vi "test_count2.vi"() -> ()   [LabVIEW 2013]
uses:
  <instrlib>/_niInstr/Basic Elements/v1/FPGA/Private/Count Down U32.vi
  <instrlib>/_niInstr/Basic Elements/v1/FPGA/niInstr Basic Elements v1 FPGA.lvlib
panel:
  out "Waveform Graph 4":i16[][](graph)
  out "Waveform Graph 3":i16[][](graph)
  out "Waveform Graph 2":u32[](graph)
  out "counting":bool
  out "output valid":bool
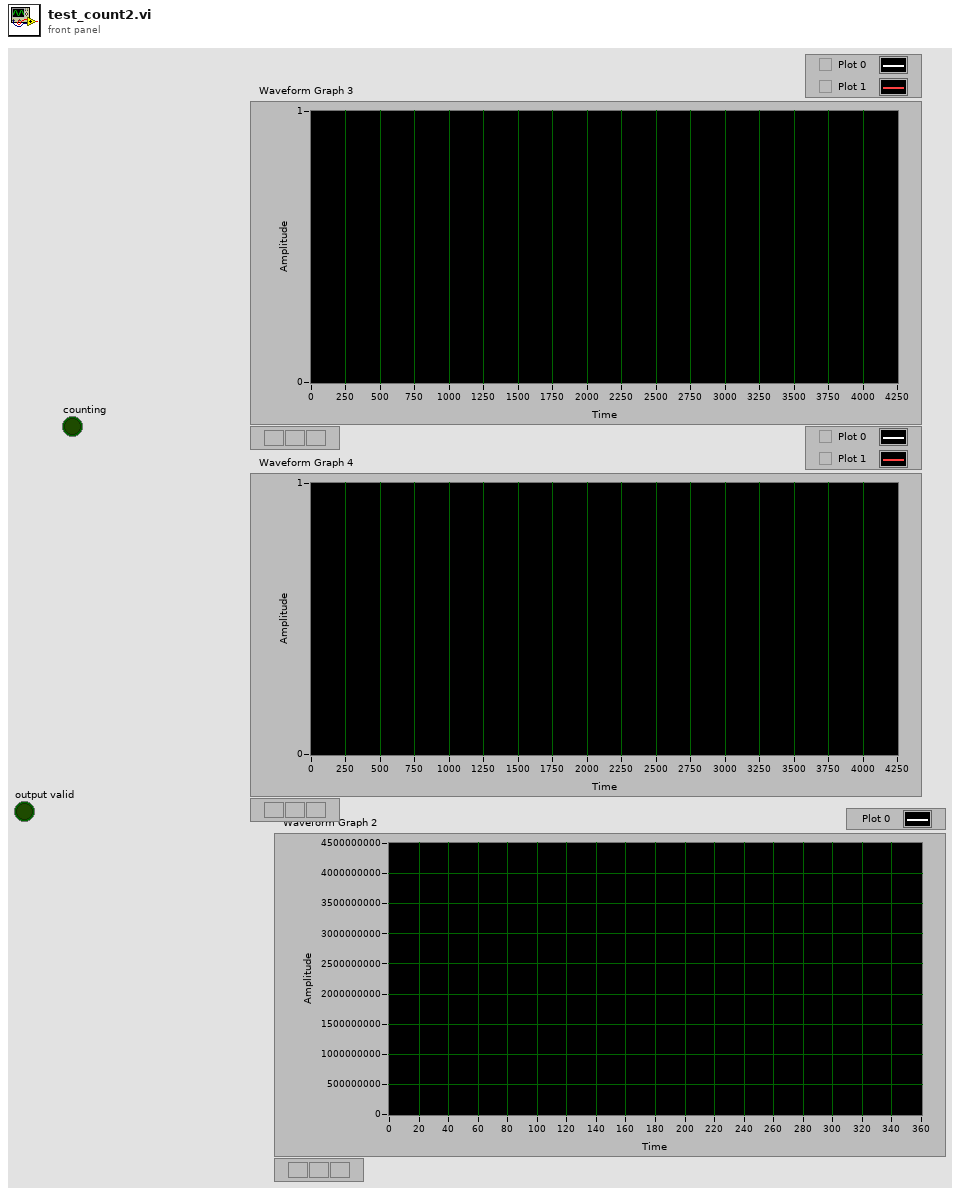
[diagram p1: front panel]
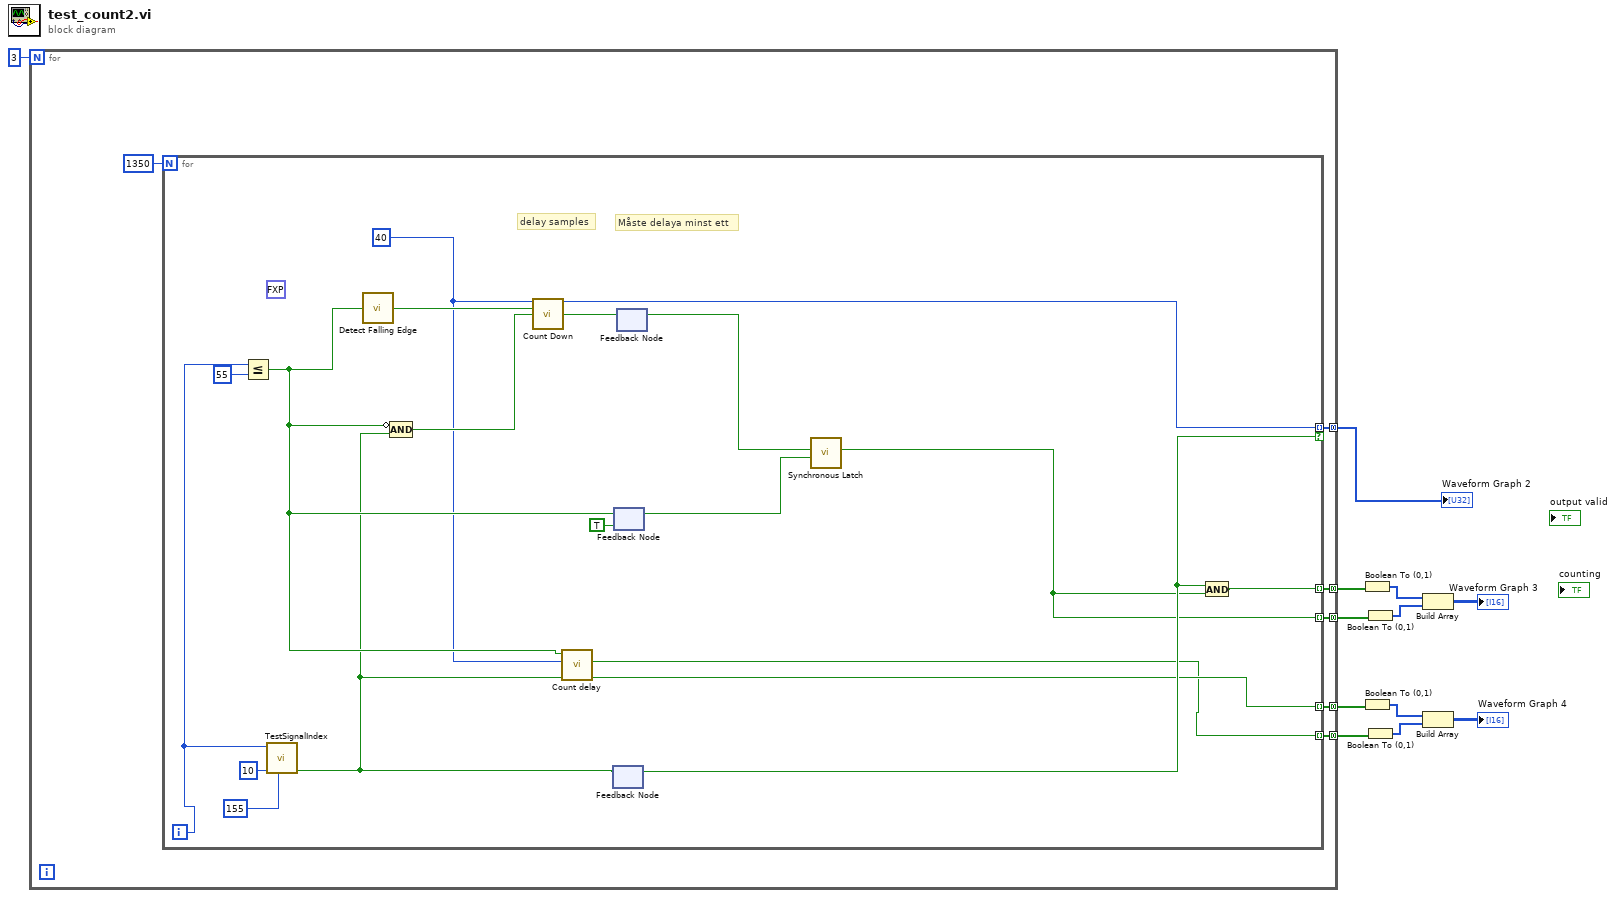
[diagram p0: block diagram]
diagram:
  n1 = for {
    N: 3 -> [_]
    tunnel: [w17] -> w12 mode=concatenating
    tunnel: [w16] -> w11 mode=concatenating
    tunnel: [w15] -> w9 mode=concatenating
    tunnel: [w13] -> w1 mode=concatenating
    tunnel: [w14] -> w2 mode=concatenating
    n2 = for {
      N: 1350 -> [_]
      tunnel: [w27] -> w17 mode=indexing
      tunnel: [w32] -> w16 mode=indexing if=w29
      tunnel: [w25] -> w15 mode=indexing
      tunnel: [w20] -> w13 mode=indexing
      tunnel: [w19] -> w14 mode=indexing
      i -> [w35]
      w22 = u32 40 ("count in")
      (unwired) fxp<+/-,16,16> 60.0 ("t")
      # "Måste delaya minst ett"
      # "delay samples"
      n3 = Less Or Equal?(x=w35, y=55) -> (x <= y?=w23:bool)
      n4 = call "TestSignalIndex.vi"("initial delay"=155, "cycles per sample"=10, "index"=w35) -> ("valid out"=w21:bool)  [unwired: 7 in, 1 out]
      n5 = call <instrlib>:"Detect Falling Edge.vi"("signal"=w23) -> ("edge detected"=w33:bool)  [unwired: 14 in]
      n6 = Compound Arithmetic op=AND(invert w23, w21) -> (w26:bool)
      n7 = call-poly <instrlib>:"Count Down.vi"("count in"=w22, "load"=w33, "decrement"=w26) -> ("count out"=w32:u32, "terminal count"=w31:bool)  [unwired: 11 in]
      n8 = call "Count delay.vi"("input valid"=w21, "Count to skip"=w22, "Reset"=w23) -> ("output valid"=w20:bool, "count done?"=w19:bool)  [unwired: 7 in]
      n9 = feedback #1() -> (w29:bool)  [unwired: 1 in]
      n10 = feedback-in #1(w21) -> ()
      n11 = feedback #2(TRUE) -> (w30:bool)
      n12 = feedback-in #2(w23) -> ()
      n13 = feedback-in #3(w31) -> ()
      n14 = feedback #3() -> (w24:bool)  [unwired: 1 in]
      n15 = call <instrlib>:"Synchronous Latch.vi"("clear"=w30, "set"=w24) -> ("out"=w25:bool)  [unwired: 9 in]
      n16 = And(x=w29, y=w25) -> (x .and. y?=w27:bool)
    }
  }
  "Waveform Graph 2" <- w11
  n17 = Boolean To (0,1)(Boolean=w12) -> (0, 1=w8:i16[])
  n18 = Boolean To (0,1)(Boolean=w1) -> (0, 1=w3:i16[])
  n19 = Boolean To (0,1)(Boolean=w9) -> (0, 1=w7:i16[])
  n20 = Boolean To (0,1)(Boolean=w2) -> (0, 1=w4:i16[])
  n21 = Build Array(w8, w7) -> (→"Waveform Graph 3":i16[][])
  n22 = Build Array(w3, w4) -> (→"Waveform Graph 4":i16[][])
